vi "GetI64.vi"(5 "format string (%.;%_20d)":string="%.;%_20d", 7 "key description":string, 8 "sections":string[](array[string]), 9 "numeric":i64, 11 "info data":string) -> (0 "sections out":string[](array[string]), 1 "key found?":bool, 2 "value":i64, 3 "info data out":string)   [LabVIEW 2020, in "infolib.lvlib"]
doc: "Add a new numeric key to Info Data string. If section exists in Info Data string, inserts key into this section."
uses:
  infolib.lvlib
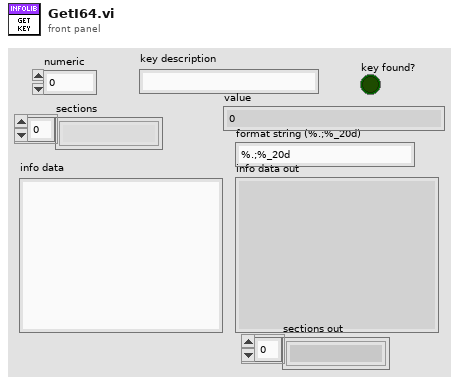
[diagram p1: front panel]
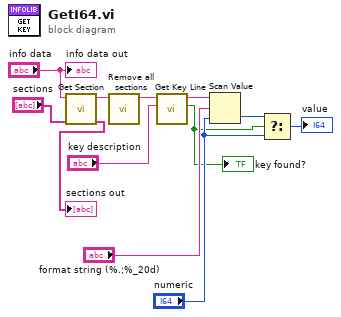
[diagram p0: block diagram]
diagram:
  n1 = call "Get Section.vi"("sections"="sections", "info data"="info data") -> ("sections out"=→"sections out":string[], "section part"=w12:string)  [unwired: 7 in, 1 out]
  n2 = call "Remove all sections.vi"("info data"=w12) -> ("info data out"=w11:string)  [unwired: 10 in]
  n3 = call "Get Key Line.vi"("key description"="key description", "info data"=w11) -> ("key found?"=w1:bool, "key value"=w7:string)  [unwired: 8 in]
  "key found?" <- w1
  n4 = Scan Value(string=w7, format string="format string (%.;%_20d)", default (0 dbl)="numeric") -> (value=w4:i64)  [unwired: 1 out]
  n5 = Select(t=w4, s=w1, f="numeric") -> (s? t:f=→"value":i64)
  "info data out" <- "info data"
